vi "DownloadRunMain.vi"(11 "Data In":T1={"Port"="", "All Code"="Hi"}) -> (0 "error out":errorcluster, 1 "Reply":string, 3 "VISA Refnum out":refnum<visa-resource-name>)   [LabVIEW 2016]
uses:
  uPythonX/PythonData.ctl
  uPythonX/uPythonX.xctl
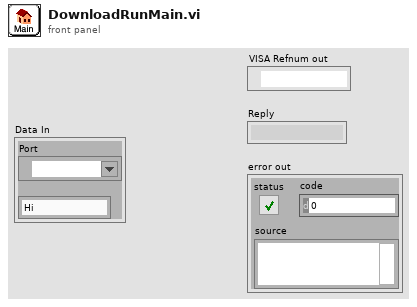
[diagram p1: front panel]
types:
  T1 = typedef "uPythonX.xctl/PythonData.ctl" = cluster{"Port":refnum<visa-resource-name>, "All Code":string}
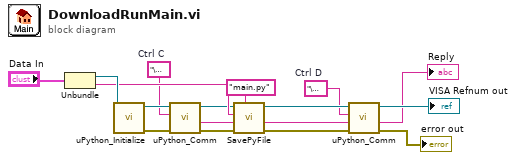
[diagram p0: block diagram]
diagram:
  w2 = "\u0003"  # Ctrl C
  w13 = "\u0004"  # Ctrl D
  n1 = Unbundle("Data In") -> ("Port"=w11:refnum<visa-resource-name>, "All Code"=w7:string)
  n2 = call "uPython_Initialize.vi"("VISA Refnum in"=w11) -> ("error out"=w6:errorcluster, "VISA Refnum out"=w5:refnum<visa-resource-name>)  [unwired: 9 in]
  n3 = call "uPython_Comm.vi"("error in (no error)"=w6, "Script"=w2, "VISA Refnum in"=w5) -> ("error out"=w4:errorcluster, "Console Out"=w1:string, "VISA out"=w3:refnum<visa-resource-name>)  [unwired: 4 in, 2 out]
  n4 = call "SavePyFile.vi"("Name"="main.py", "error in"=w4, "Console In"=w1, "Python Code"=w7, "VISA in"=w3) -> ("error out"=w15:errorcluster, "Reply"=w10:string, "VISA out"=w17:refnum<visa-resource-name>)  [unwired: 4 in]
  n5 = call "uPython_Comm.vi"("error in (no error)"=w15, "Console In"=w10, "Script"=w13, "VISA Refnum in"=w17) -> ("error out"=→"error out":errorcluster, "Console Out"=→"Reply":string, "VISA out"=→"VISA Refnum out":refnum<visa-resource-name>)  [unwired: 3 in, 2 out]
